vi "FGV_Pattern.vi"(4 "Opción":enum16{"Write", "Read"}(ring), 5 "Error In":errorcluster) -> (19 "Error Out":errorcluster)   [LabVIEW 2013]
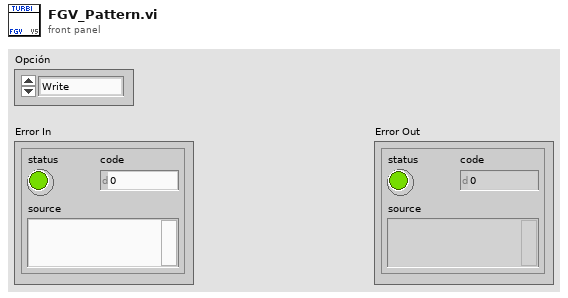
[diagram p1: front panel]
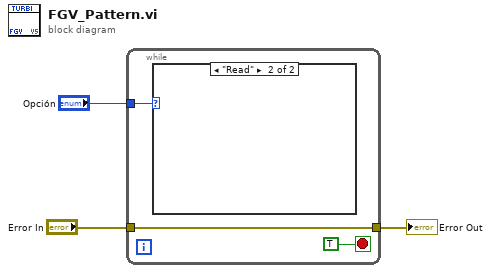
[diagram p0: block diagram]
diagram:
  n1 = while {
    tunnel: "Opción" -> [w5]
    tunnel: [w4] -> w2
    tunnel: "Error In" -> [w4]
    stop <- TRUE stop-if-true
    n2 = case shown="\"Read\"" w5 {
      frame "Write", Default {
      }
      frame "Read" {
      }
    }
  }
  "Error Out" <- w2
